vi "Destroy User Events.vi"(8 "error in (no error)":errorcluster, 11 "Helper Loop in":refnum<class "Helper Loop.lvclass">) -> (0 "error out":errorcluster, 3 "Helper Loop out":refnum<class "Helper Loop.lvclass">)   [LabVIEW 2024, in "Helper Loop.lvlib" / "Helper Loop.lvclass"]
uses:
  Helper Loop.lvclass
  Helper Loop.lvclass/Helper Loop.ctl
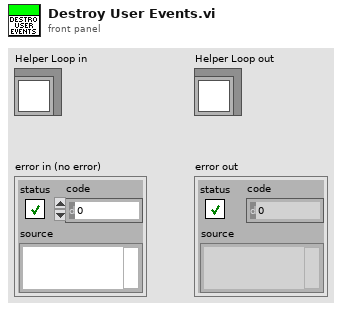
[diagram p1: front panel]
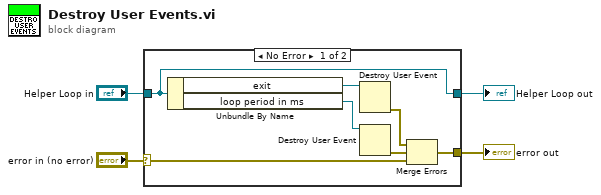
[diagram p0: block diagram]
diagram:
  n1 = case shown="No Error" "error in (no error)" {
    selector: "error in (no error)" -> [w5 w13]
    tunnel: [w11 w12] -> w2
    tunnel: "Helper Loop in" -> [w11 w12]
    tunnel: [w6 w13] -> w1
    frame No Error {
      n2 = Unbundle By Name(w11) -> ("exit"=w10:refnum<user-event>, "loop period in ms"=w9:refnum<user-event>)
      n3 = Destroy User Event(user event=w10) -> (error out=w8:errorcluster)  [unwired: 1 in]
      n4 = Destroy User Event(user event=w9) -> (error out=w7:errorcluster)  [unwired: 1 in]
      n5 = Merge Errors(w8, w7, w5) -> (w6:errorcluster)
    }
    frame Error {
    }
  }
  "error out" <- w1
  "Helper Loop out" <- w2
